vi "initialize Session Data.vi"(0 "Session in":refnum<class "Result Data Mgr.lvclass">, 11 "error in":errorcluster) -> (4 "Session out":refnum<class "Result Data Mgr.lvclass">, 15 "error out":errorcluster)   [LabVIEW 2018, in "Result Data Mgr.lvclass"]
uses:
  Result Data Mgr.lvclass
  Typedefs/GRR Result.ctl
  Result Data Mgr.lvclass/Result Data Mgr.ctl
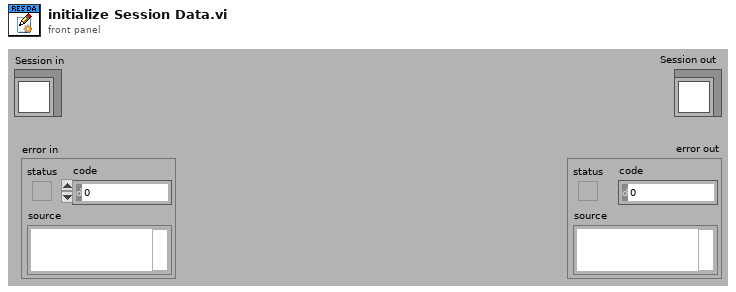
[diagram p1: front panel]
types:
  T1 = typedef "Result Data Mgr.lvclass/GRR Result.ctl" = cluster{"Test Name":string, "Parts #":u8, "Appraiser #":u8, "Trial #":u8, "Percent AV":dbl, "Percent EV":dbl, "Percent GRR":dbl}
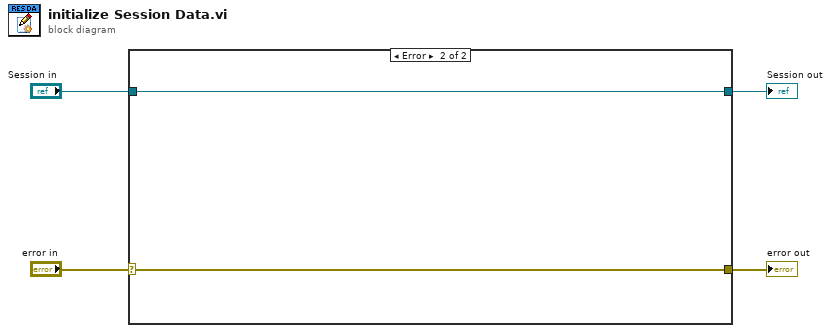
[diagram p0: block diagram]
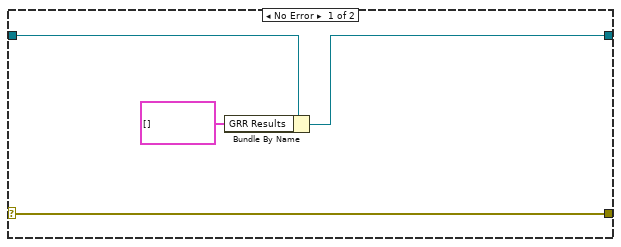
[diagram p2: hidden frame]
diagram:
  n1 = case shown="Error" "error in" {
    selector: "error in" -> [w5 w9]
    tunnel: "Session in" -> [w8 w10]
    tunnel: [w6 w10] -> w2
    tunnel: [w5 w9] -> w1
    frame No Error {
      n2 = Bundle By Name(cluster=w8, "GRR Results"=T1[] []) -> (w6:refnum<class "Result Data Mgr.lvclass">)
    }
    frame Error {
    }
  }
  "error out" <- w1
  "Session out" <- w2
